vi "Pre Launch Init.vi"(11 "Measurement gg in":refnum<class "Measurement gg.lvclass">) -> (0 "error out":errorcluster, 3 "Measurement gg out":refnum<class "Measurement gg.lvclass">)   [LabVIEW 2020, in "Measurement gg.lvlib" / "Measurement gg.lvclass"]
doc: "(<B>Filename</B>: Actor Framework.lvlib:Actor.lvclass:Pre Launch Init.vi)\n\nDefines behavior that occurs after the Launch Nested Actor method is invoked but before the actor's Actor Core method begins running.\n\nBy default, this method does nothing. A descendant class may override it to define behavior."
uses:
  Measurement gg.lvclass
  Measurement gg.lvclass/Measurement gg.ctl
  <vilib>/ActorFramework/Actor/Actor.lvclass
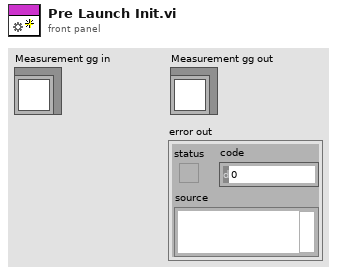
[diagram p1: front panel]
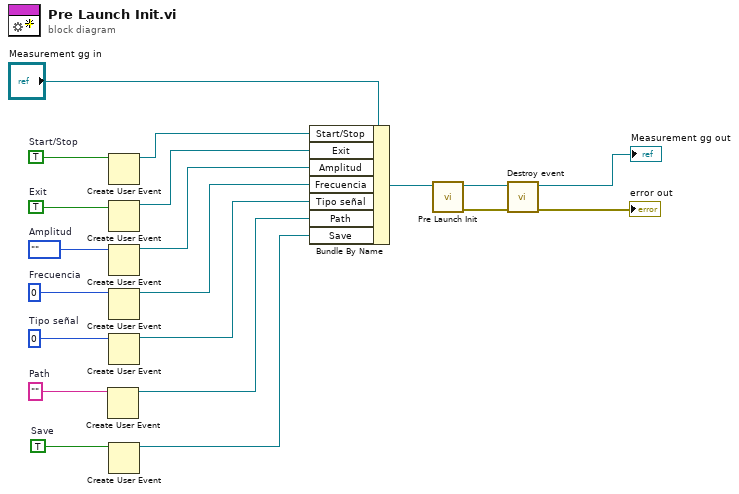
[diagram p0: block diagram]
diagram:
  w2 = TRUE  # Save
  w5 = ""  # Path
  w20 = enum16{""}.""  # Amplitud
  w16 = 0  # Tipo señal
  w17 = 0  # Frecuencia
  w18 = TRUE  # Exit
  w19 = TRUE  # Start/Stop
  n1 = Create User Event(user event datatype=w5) -> (user event=w3:refnum<user-event>)  [unwired: 1 in, 1 out]
  n2 = Create User Event(user event datatype=w19) -> (user event=w13:refnum<user-event>)  [unwired: 1 in, 1 out]
  n3 = Create User Event(user event datatype=w18) -> (user event=w12:refnum<user-event>)  [unwired: 1 in, 1 out]
  n4 = Create User Event(user event datatype=w20) -> (user event=w11:refnum<user-event>)  [unwired: 1 in, 1 out]
  n5 = Create User Event(user event datatype=w17) -> (user event=w4:refnum<user-event>)  [unwired: 1 in, 1 out]
  n6 = Create User Event(user event datatype=w16) -> (user event=w10:refnum<user-event>)  [unwired: 1 in, 1 out]
  n7 = Create User Event(user event datatype=w2) -> (user event=w1:refnum<user-event>)  [unwired: 1 in, 1 out]
  n8 = Bundle By Name(cluster="Measurement gg in", "Start/Stop"=w13, "Exit"=w12, "Amplitud"=w11, "Frecuencia"=w4, "Tipo señal"=w10, "Path"=w3, "Save"=w1) -> (w15:refnum<class "Measurement gg.lvclass">)
  n9 = call-parent "Pre Launch Init.vi"("Actor in"=w15) -> ("error out"=w9:errorcluster, "Actor out"=w6:refnum<class "Measurement gg.lvclass">)  [unwired: 9 in]
  n10 = call "Destroy event.vi"("error in (no error)"=w9, "Measurement gg in"=w6) -> ("error out"=→"error out":errorcluster, "Measurement gg out"=→"Measurement gg out":refnum<class "Measurement gg.lvclass">)  [unwired: 8 in]
